vi "TDMS Write.vi"(7 "Channel Name":string, 8 "error in (no error)":errorcluster, 9 "Group Name":string, 10 "TDMS in":refnum<k34>, 11 "Cluster Array in":refnum<class "Cluster Array.lvclass">) -> (0 "error out":errorcluster, 2 "TDMS Out":refnum<k34>)   [LabVIEW 2020, in "Data.lvlib" / "Cluster Array.lvclass"]
doc: "Write Generic Data to a TDMS file."
uses:
  Cluster Array.lvclass
  Cluster Array.lvclass/Cluster Array.ctl
  Cluster/Cluster.lvclass
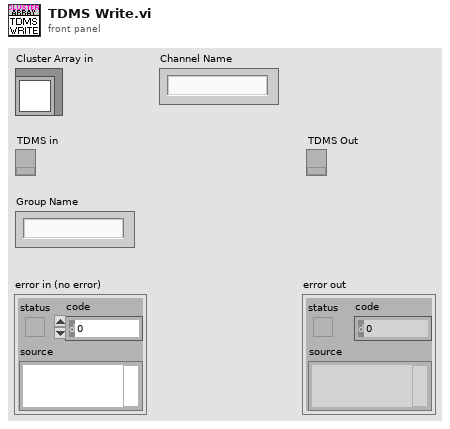
[diagram p1: front panel]
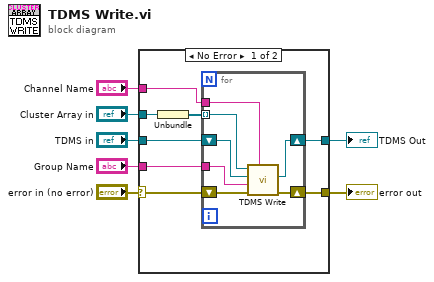
[diagram p0: block diagram]
diagram:
  n1 = case shown="No Error" "error in (no error)" {
    selector: "error in (no error)" -> [w9 w23]
    tunnel: [w8 w23] -> w1
    tunnel: "TDMS in" -> [w11 w24]
    tunnel: [w10 w24] -> w6
    tunnel: "Channel Name" -> [w13 _]
    tunnel: "Group Name" -> [w12 _]
    tunnel: "Cluster Array in" -> [w15 _]
    frame No Error {
      n2 = Unbundle(w15) -> (w14:refnum<class "Cluster.lvclass">[])
      n3 = for {
        tunnel: w14 -> [w22] mode=indexing
        tunnel: w13 -> [w21]
        tunnel: w12 -> [w20]
        shift-right: [w18] -> w10
        shift-left: w11 -> [w19]
        shift-right: [w16] -> w8
        shift-left: w9 -> [w17]
        n4 = call-dynamic "TDMS Write.vi"("Channel Name"=w21, "error in (no error)"=w17, "Group Name"=w20, "TDMS in"=w19, "Cluster in"=w22) -> ("error out"=w16:errorcluster, "TDMS Out"=w18:refnum<k34>)  [unwired: 5 in]
      }
    }
    frame Error {
    }
  }
  "error out" <- w1
  "TDMS Out" <- w6
